vi "Add Elements to Array Channel.vi"(7 "array element GUID":string, 8 "error in (no error)":errorcluster, 10 "array elements":T2[](array[typedef]), 11 "array refnum in":T1 format="%.0x") -> (0 "error out":errorcluster, 2 "channel refnums":T1[](array[typedef]) format="%.0x", 3 "array refnum out":T1 format="%.0x")   [LabVIEW 2018, in "Instrument Addon Scripting API.lvlib"]
doc: "Adds channels under the Data Array section provided as reference input."
uses:
  Instrument Addon Scripting API.lvlib
  <vilib>/NI Veristand/Custom Device API/Custom Device Item Ref.ctl
  TypeDefs/Array Element.ctl
  <vilib>/NI Veristand/Custom Device API/Custom Device Channel Type.ctl
  <vilib>/NI Veristand/Custom Device API/Custom Device Channel.ctl
  <vilib>/NI Veristand/Custom Device API/Custom Device API.lvlib
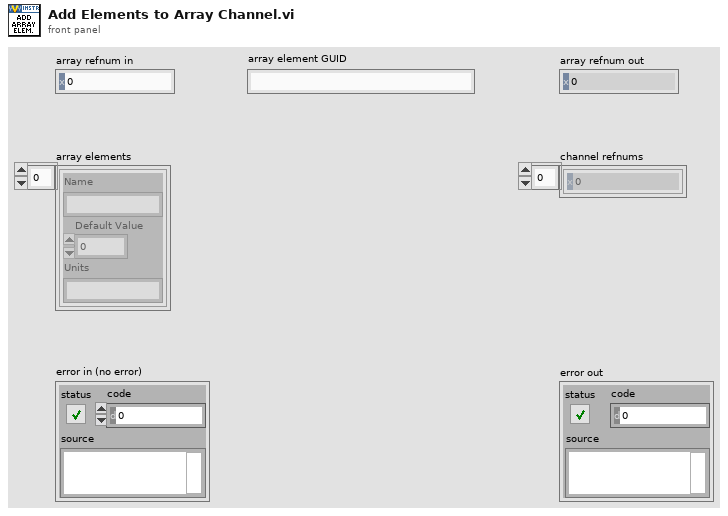
[diagram p1: front panel]
types:
  T1 = typedef "Custom Device API.lvlib/Custom Device Item Ref.ctl" = u64
  T2 = typedef "Instrument Addon Scripting API.lvlib/Array Element.ctl" = cluster{"Name":string, "Default Value":dbl, "Units":string}
  T3 = typedef "Custom Device API.lvlib/Custom Device Channel Type.ctl" = enum16{"Input", "Output"}
  T4 = typedef "Custom Device API.lvlib/Custom Device Channel.ctl" = cluster{"Type":T3, "Units":string, "Default Value":dbl, "Faultable":bool, "Scalable":bool}
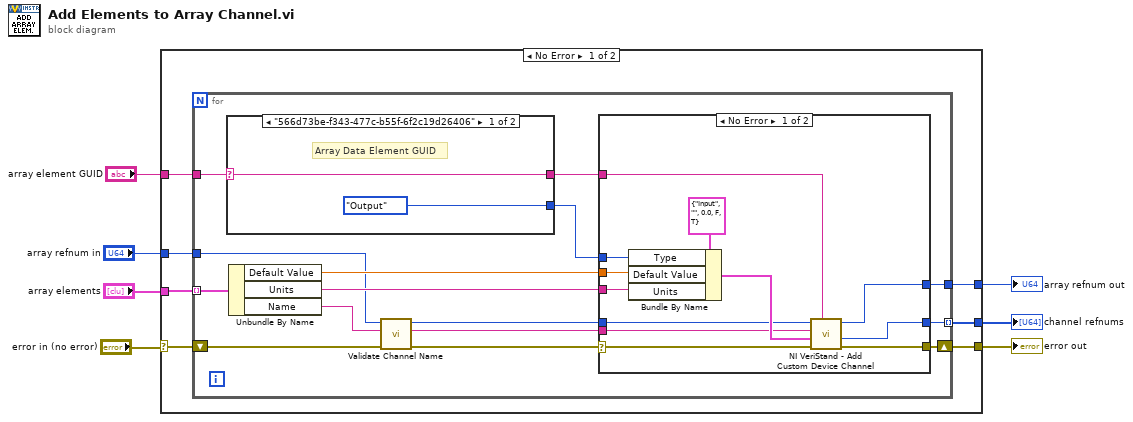
[diagram p0: block diagram]
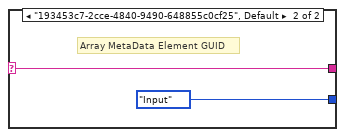
[diagram p2: hidden frame]
diagram:
  n1 = case shown="No Error" "error in (no error)" {
    selector: "error in (no error)" -> [w12 w49]
    tunnel: [w14 w49] -> w7
    tunnel: "array refnum in" -> [w13 w48]
    tunnel: "array elements" -> [w10 _]
    tunnel: [w11 _] -> w4
    tunnel: [w9 w48] -> w3
    tunnel: "array element GUID" -> [w8 _]
    frame No Error {
      n2 = for {
        shift-right: [w29] -> w14
        shift-left: w12 -> [w20]
        tunnel: w13 -> [w18]
        tunnel: w10 -> [w28] mode=indexing
        tunnel: [w25] -> w11 mode=indexing
        tunnel: [w24] -> w9
        tunnel: w8 -> [w17]
        n3 = case shown="\"566d73be-f343-477c-b55f-6f2c19d26406\"" w17 {
          selector: w17 -> [w30 w32]
          tunnel: [Custom_Device_Channel_Type."Output" ("Type") Custom_Device_Channel_Type."Input" ("Type")] -> w16
          tunnel: [w30 w32] -> w15
          frame "566d73be-f343-477c-b55f-6f2c19d26406" {
            # "Array Data Element GUID"
          }
          frame "193453c7-2cce-4840-9490-648855c0cf25", Default {
            # "Array MetaData Element GUID"
          }
        }
        n4 = Unbundle By Name(w28) -> ("Default Value"=w27:dbl, "Units"=w26:string, "Name"=w19:string)
        n5 = call "Validate Channel Name.vi"("error in (no error)"=w20, "Name In"=w19, "Refnum In"=w18) -> ("error out"=w21:errorcluster, "Name Out"=w22:string, "Refnum Out"=w23:T1)  [unwired: 6 in]
        n6 = case shown="No Error" w21 {
          selector: w21 -> [w39 w47]
          tunnel: [w45 w47] -> w29
          tunnel: w23 -> [w43 w46]
          tunnel: w27 -> [w42 _]
          tunnel: w26 -> [w41 _]
          tunnel: w22 -> [w40 _]
          tunnel: [w38 _] -> w25
          tunnel: [w37 w46] -> w24
          tunnel: w16 -> [w35 _]
          tunnel: w15 -> [w34 _]
          frame No Error {
            n7 = Bundle By Name(cluster=T4 {"Type"=enum."Input", "Units"="", "Default Value"=0.0, "Faultable"=FALSE, "Scalable"=TRUE} ("Channel"), "Type"=w35, "Default Value"=w42, "Units"=w41) -> (w44:T4)
            n8 = call <vilib>:"NI VeriStand - Add Custom Device Channel.vi"("GUID (Default Channel)"=w34, "error in (no error)"=w39, "Channel"=w44, "Channel Name"=w40, "Parent Ref in"=w43) -> ("error out"=w45:errorcluster, "Channel Ref"=w38:T1, "Parent Ref out"=w37:T1)  [unwired: 3 in, 1 out]
          }
          frame Error {
          }
        }
      }
    }
    frame Error {
    }
  }
  "error out" <- w7
  "channel refnums" <- w4
  "array refnum out" <- w3
